vi "Gmsg_PS_Subscriber.vi"() -> ()   [LabVIEW 2015]
uses:
  source/actor/Message/Base/FTW-Message.lvclass
  source/actor/Subscriber/FTW-Subscriber.lvclass
panel:
  in  "Connection":string(combo)="lvq://someLVQconnection"
  out "Body":string
  out "Header":string
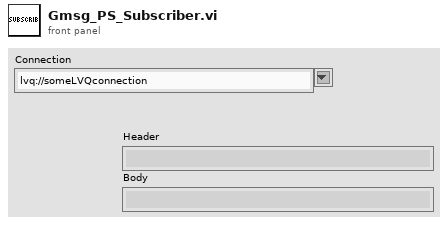
[diagram p1: front panel]
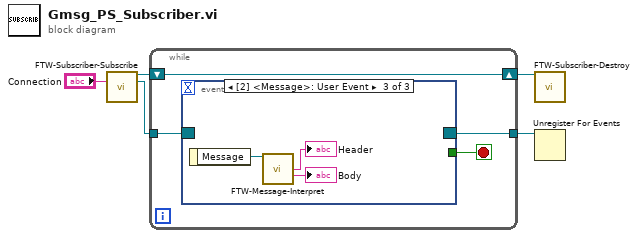
[diagram p0: block diagram]
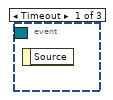
[diagram p2: hidden frame]
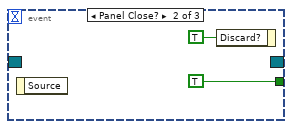
[diagram p3: hidden frame]
diagram:
  n1 = call "FTW-Subscriber-Subscribe.vi"("Addresses"="Connection") -> ("FTW-Subscription Out"=w4:refnum<class "FTW-Subscriber.lvclass">, "Subscriber Registration"=w3:refnum<event-registration>)  [unwired: 12 in, 1 out]
  n2 = while {
    tunnel: w3 -> [w8]
    tunnel: [w7] -> w5
    shift-right: [w6] -> w2
    shift-left: w4 -> [w6]
    stop <- w9 stop-if-true
    n3 = event shown="[2] <Message>: User Event" {
      selector: w8 -> [_ _ _]
      dyn-events: [_ _ _] -> w7
      timeout: _ -> [_ _ _]
      tunnel: [_ TRUE _] -> w9
      event Timeout {
        n4 = event-data() -> ()  [unwired: 1 in, 1 out]
      }
      event Panel Close? {
        n5 = event-data() -> ()  [unwired: 1 in, 1 out]
        n6 = event-data("Discard?"=TRUE) -> ()  [unwired: 1 in, 1 out]
      }
      event User Event {
        n7 = event-data() -> ("Message"=w14:refnum<class "FTW-Message.lvclass">)  [unwired: 1 in]
        n8 = call-dynamic "FTW-Message-Interpret.vi"("FTW Message"=w14) -> ("Message Header"=→"Header":string, "Message Body"=→"Body":string)  [unwired: 10 in, 3 out]
      }
    }
  }
  n9 = call "FTW-Subscriber-Destroy.vi"("FTW-Subscription In"=w2) -> ()  [unwired: 14 in, 1 out]
  n10 = Unregister For Events(event registration refnum=w5) -> ()  [unwired: 1 in, 1 out]
